vi "initialize servers.vi"(8 "error in (no error)":errorcluster, 11 "Channel in":refnum<class "Channel.lvclass">) -> (0 "error out":errorcluster, 3 "Channel out":refnum<class "Channel.lvclass">)   [LabVIEW 2018, in "Channel.lvclass"]
uses:
  Channel.lvclass
  Server/Server.lvclass
  Server/Server.lvclass/Server.ctl
  Channel.lvclass/Channel.ctl
panel:
  in  "Server.lvclass":refnum<class "Server.lvclass">
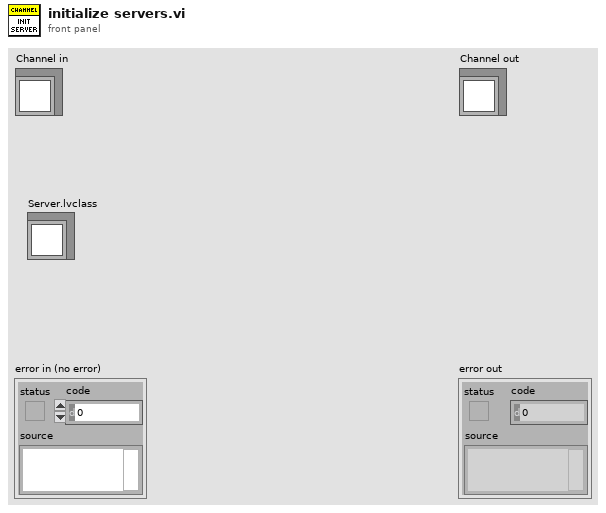
[diagram p1: front panel]
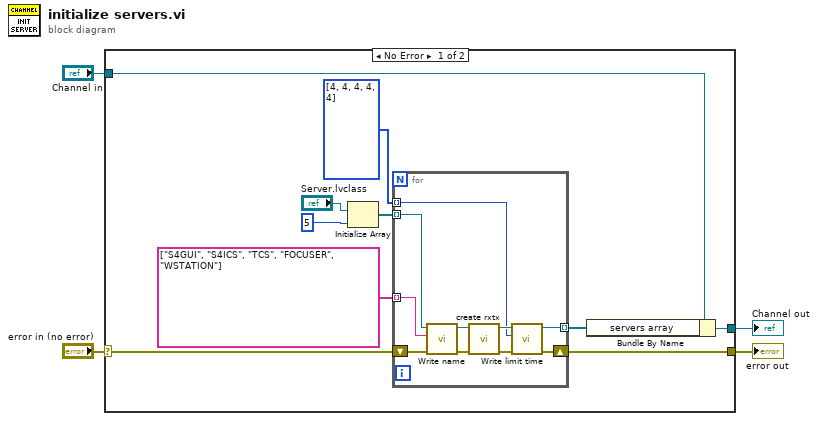
[diagram p0: block diagram]
diagram:
  n1 = case shown="No Error" "error in (no error)" {
    selector: "error in (no error)" -> [w8 w26]
    tunnel: [w14 w26] -> w2
    tunnel: [w13 w25] -> w1
    tunnel: "Channel in" -> [w6 w25]
    frame No Error {
      n2 = Initialize Array("Server.lvclass", 5 ("dimension size")) -> (w12:refnum<class "Server.lvclass">[])
      n3 = for {
        shift-right: [w20] -> w14
        shift-left: w8 -> [w19]
        tunnel: w12 -> [w17] mode=indexing
        tunnel: [w21] -> w10 mode=indexing
        tunnel: string[] ["S4GUI", "S4ICS", "TCS", "FOCUSER", "WSTATION"] -> [w15] mode=indexing
        tunnel: u16[] [4, 4, 4, 4, 4] -> [w22] mode=indexing
        n4 = call-dynamic "Write name.vi"("error in (no error)"=w19, "name"=w15, "Server in"=w17) -> ("error out"=w18:errorcluster, "Server out"=w16:refnum<class "Server.lvclass">)  [unwired: 7 in]
        n5 = call "create rxtx.vi"("error in (no error)"=w18, "Server in"=w16) -> ("error out"=w24:errorcluster, "Server out"=w23:refnum<class "Server.lvclass">)  [unwired: 8 in]
        n6 = call "Write limit time.vi"("error in (no error)"=w24, "limit time"=w22, "Server in"=w23) -> ("error out"=w20:errorcluster, "Server out"=w21:refnum<class "Server.lvclass">)  [unwired: 7 in]
      }
      n7 = Bundle By Name(cluster=w6, "servers array"=w10) -> (w13:refnum<class "Channel.lvclass">)
    }
    frame Error {
    }
  }
  "error out" <- w2
  "Channel out" <- w1
